vi "Prepare Update Command.vi"(8 "Error In (no error)":errorcluster, 10 "Record":variant) -> (0 "Error Out":errorcluster, 2 "Insert SQL Command":string)   [LabVIEW 2023, in "SQLite DB Operator.lvclass"]
uses:
  <vilib>/JDP Science/JDP Science Common Utilities/Trim Whitespace__JDP.vi
  <userlib>/_OpenG.lib/array/array.llb/Search 1D Array (String)__ogtk.vi
  SQLite DB Operator.lvclass
  SQLite DB Operator.lvclass/SQLite DB Operator.ctl
  <vilib>/Utility/Data Type/NI_Data Type.lvlib
  <vilib>/drjdpowell/SQLite Library/SQLite.lvlib
  <userlib>/_OpenG.lib/array/array.llb/Delete Elements from 1D Array (String)__ogtk.vi
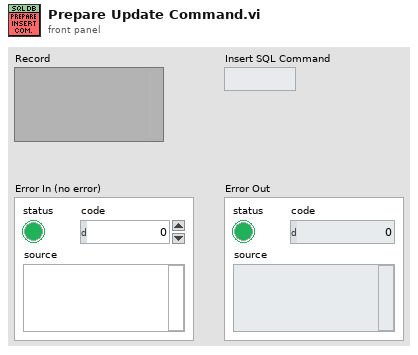
[diagram p1: front panel]
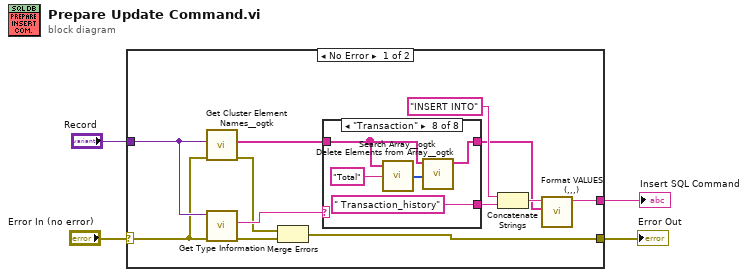
[diagram p0: block diagram]
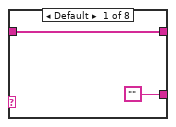
[diagram p2: hidden frame]
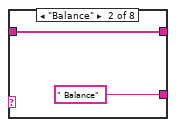
[diagram p3: hidden frame]
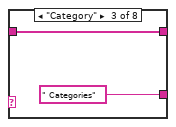
[diagram p4: hidden frame]
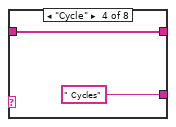
[diagram p5: hidden frame]
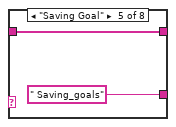
[diagram p6: hidden frame]
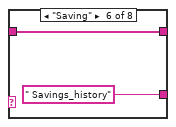
[diagram p7: hidden frame]
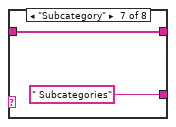
[diagram p8: hidden frame]
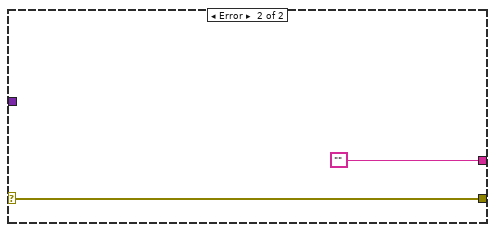
[diagram p9: hidden frame]
diagram:
  n1 = case shown="No Error" "Error In (no error)" {
    selector: "Error In (no error)" -> [w6 w37]
    tunnel: [w14 w37] -> w4
    tunnel: [w11 ""] -> w3
    tunnel: "Record" -> [w7 _]
    frame No Error {
      n2 = call <userlib>:"Get Cluster Element Names__ogtk.vi"("error in (no error)"=w6, "Cluster"=w7) -> ("error out"=w9:errorcluster, "Element Names"=w8:string[])  [unwired: 8 in]
      n3 = call <vilib>:"Get Type Information.vi"("error in (no error)"=w6, "variant"=w7) -> ("error out"=w10:errorcluster, "name"=w16:string)  [unwired: 5 in, 3 out]
      n4 = Merge Errors(w9, w10) -> (w14:errorcluster)
      n5 = case shown="\"Transaction\"" w16 {
        tunnel: ["" " Balance" ("string") " Categories" ("string") " Cycles" ("string") " Saving_goals" ("string") " Savings_history" ("string") " Subcategories" ("string") " Transaction_history" ("string")] -> w12
        tunnel: w8 -> [w17 w19 w21 w23 w25 w27 w29 w32]
        tunnel: [w17 w19 w21 w23 w25 w27 w29 w31] -> w5
        frame Default {
        }
        frame "Balance" {
        }
        frame "Category" {
        }
        frame "Cycle" {
        }
        frame "Saving Goal" {
        }
        frame "Saving" {
        }
        frame "Subcategory" {
        }
        frame "Transaction" {
          n6 = call-poly <userlib>:"Search Array__ogtk.vi"("Array"=w32, "Element Data"="Total") -> ("Indices of Elements"=w33:i32[])  [unwired: 7 in]
          n7 = call-poly <userlib>:"Delete Elements from Array__ogtk.vi"("indices"=w33, "array"=w32) -> ("array w/ subset deleted"=w31:string[])  [unwired: 8 in, 1 out]
        }
      }
      n8 = Concatenate Strings("INSERT INTO", w12) -> (w13:string)
      n9 = call <vilib>:"Format VALUES (,,,).vi"("Column Names"=w5, "partial SQL"=w13) -> ("SQL"=w11:string)  [unwired: 9 in]
    }
    frame Error {
    }
  }
  "Error Out" <- w4
  "Insert SQL Command" <- w3
